vi "Update Graphs_Brass.vi"(0 "Select Graph":T8=enum."Temperature (F)", 2 "appended array":refnum<vi>[](array[refnum]), 5 "ERD Graph  Ind 2":T7, 7 "All_Bundled_Data_Brass":T1, 11 "Error In":errorcluster) -> (4 "All Loads":u16[][](graph), 12 "ERD 3":dbl(graph), 13 "ERD 2":dbl(graph), 14 "ERD 1":dbl(graph), 15 "Error Out":errorcluster)   [LabVIEW 2016]
doc: "This VI displays (makes visable) the corresponding graph based on user selection, as well as updates the values of the graphs with current data."
uses:
  type defs2/Select _Graph_Brass.ctl
  type defs2/All_Bundled_Data_Brass.ctl
  Laundry Tool 1.0 Support/type defs/Version.ctl
  type defs2/ERD_Always_Show_Brass.ctl
  type defs2/CSV_File_String_Arrays.ctl
  type defs2/Fault Table Array.ctl
  Laundry Tool 1.0 Support/type defs/Fault_Table_Info.ctl
panel:
  # "Software Version"
  # "UI"
  # "MC"
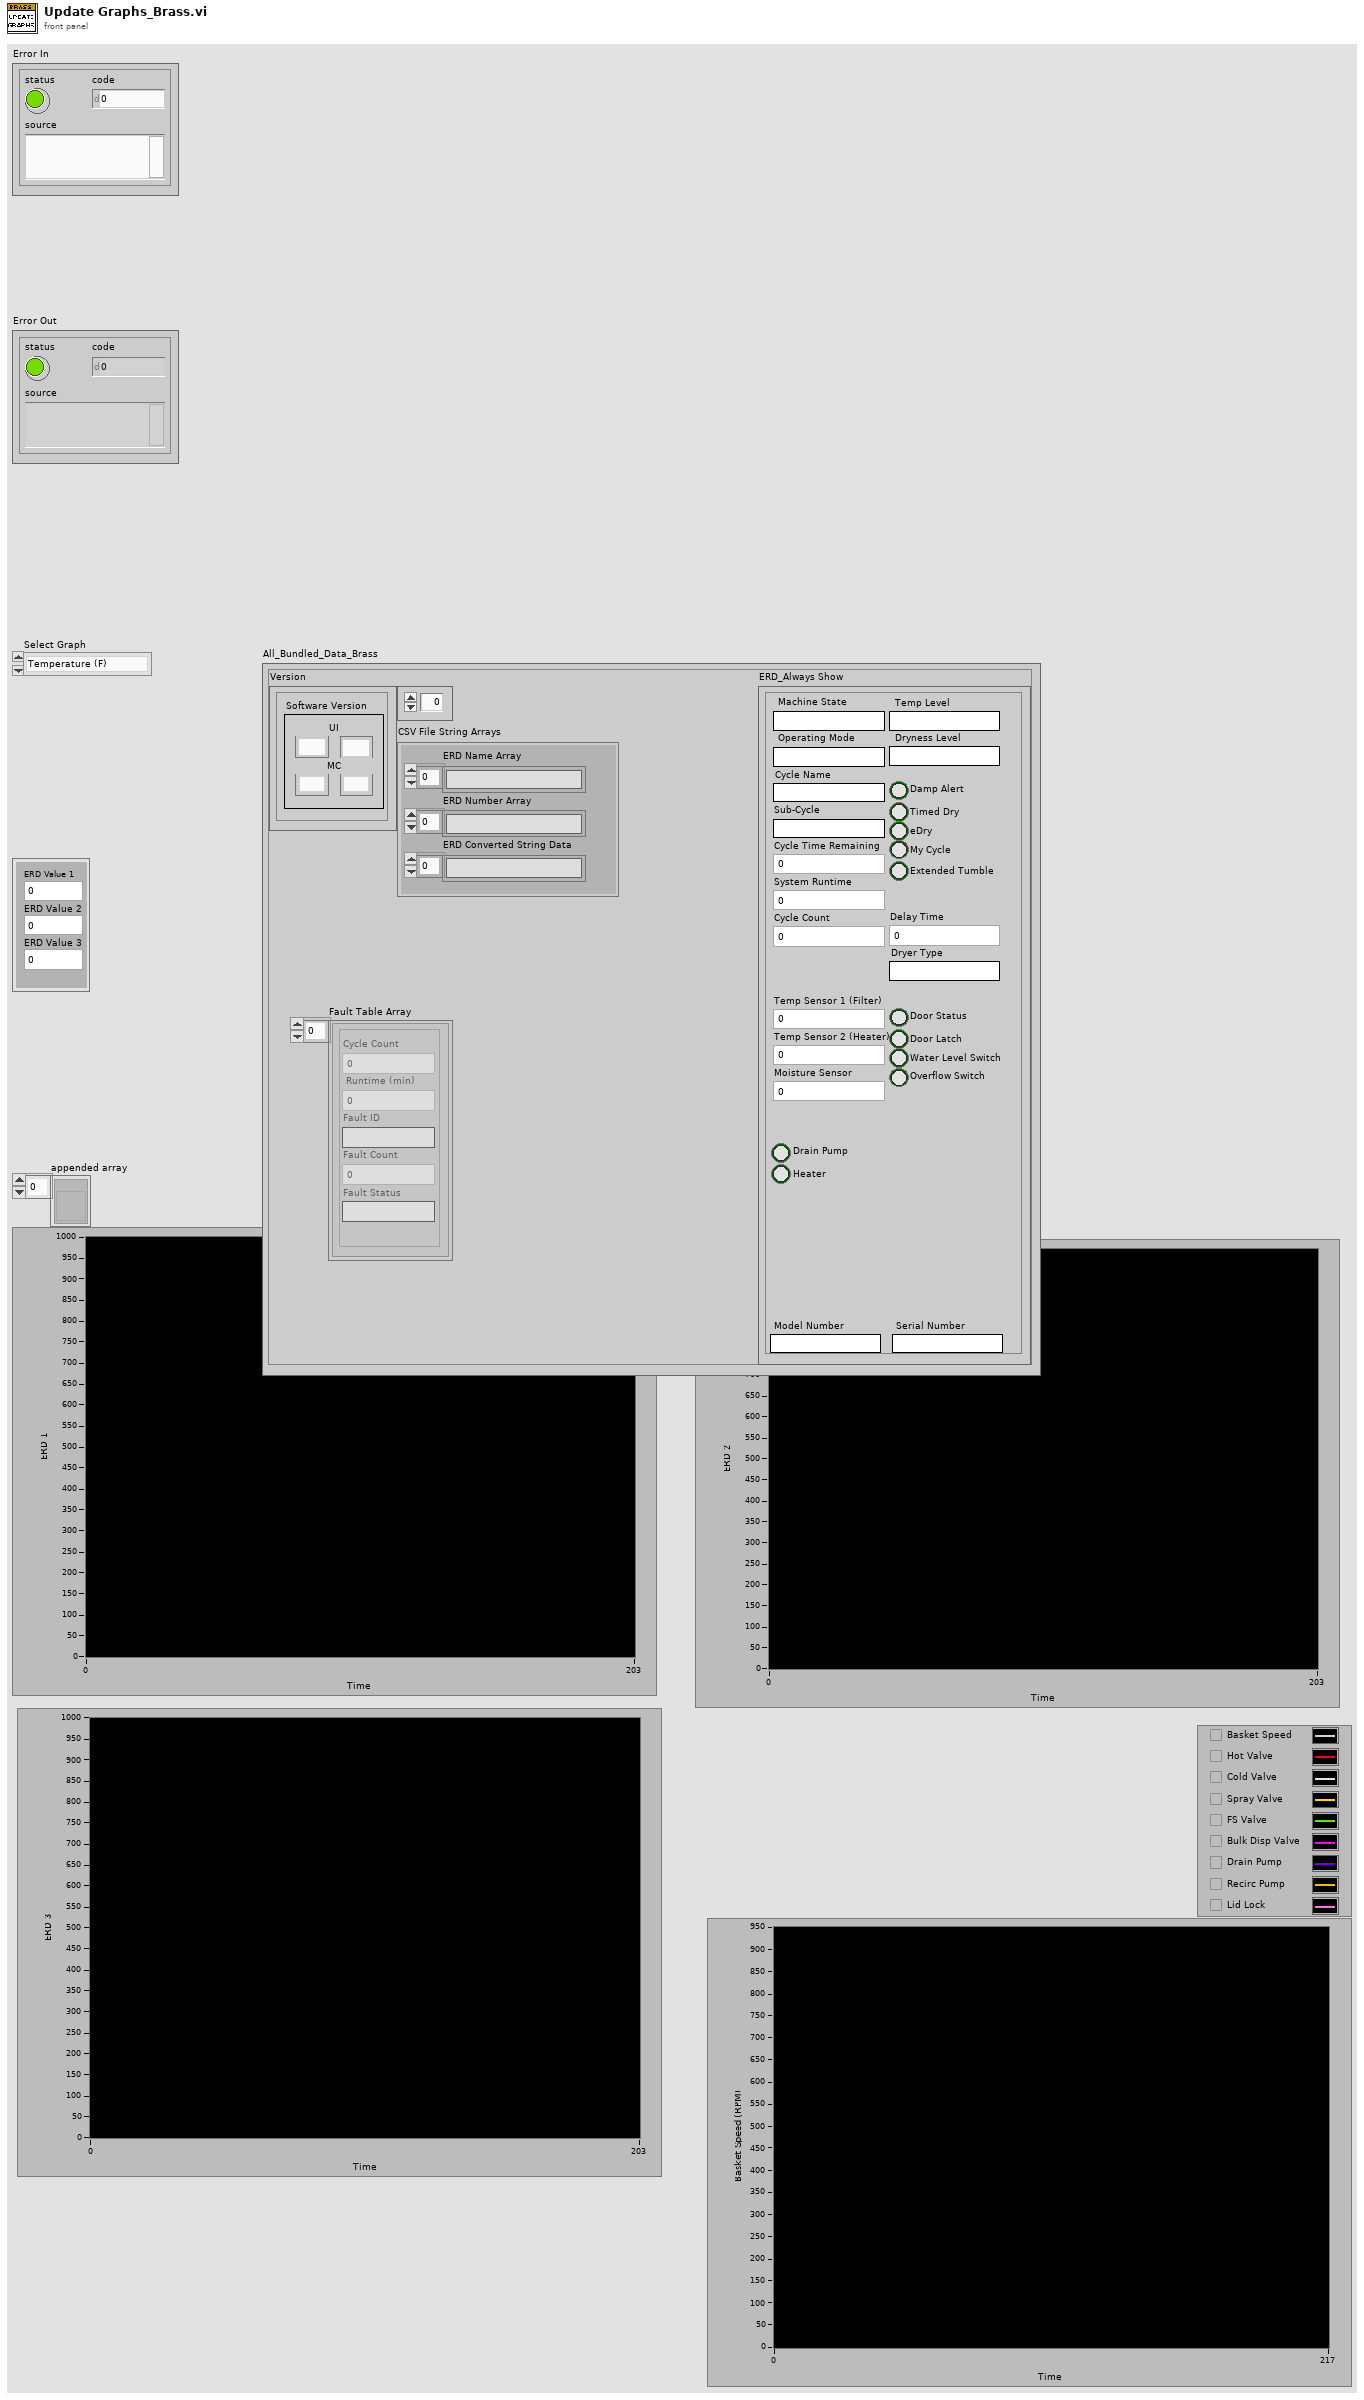
[diagram p1: front panel]
types:
  T1 = typedef "All_Bundled_Data_Brass.ctl" = cluster{"Version":T2, "ERD_Always Show":T3, "Personality Set":u8, "CSV File String Arrays":T4, "Fault Table Array ":T5}
  T2 = typedef "Version.ctl" = cluster{"Critical Major":string, "Critical Minor":string, "Non-Critical Minor":string, "Non-Critical Major":string}
  T3 = typedef "ERD_Always_Show_Brass.ctl" = cluster{"Machine State":string, "Cycle Count":u32, "Dryness Level":string, "Temp Level":string, "Delay Time":u16, "Sub-Cycle":string, "Cycle Name":string, "Model Number":string, "Serial Number":string, "System Runtime":u32, "Cycle Time Remaining":u16, "Operating Mode":string, "Temp Sensor 1 (Filter)":u16, "Drain Pump":bool, "Water Level Switch":bool, "Overflow Switch":bool, "Door Status":bool, "Door Latch":bool, "Heater":bool, "Temp Sensor 2 (Heater)":u16, "Moisture Sensor":u16, "Dryer Type":string, "eDry":bool, "Damp Alert":bool, "Timed Dry":bool, "My Cycle":bool, "Extended Tumble":bool}
  T4 = typedef "CSV_File_String_Arrays.ctl" = cluster{"ERD Number Array":string[], "ERD Name Array":string[], "ERD Converted String Data":string[]}
  T5 = typedef "Fault Table Array.ctl" = T6[]
  T6 = typedef "Fault_Table_Info.ctl" = cluster{"Cycle Count":u32, " Runtime (min) ":u32, "Fault Status":string, "Fault ID":string, "Fault Count":u16}
  T7 = cluster{"ERD Value 1":dbl, "ERD Value 2":dbl, "ERD Value 3":dbl}
  T8 = typedef "Select _Graph_Brass.ctl" = enum16{"All Loads", "ERD 1", "ERD 2", "ERD 3", "Temperature (F)", "Basket Speed (RPM)", "Tub Volume (Gal)", "Pressure (in H2O)", "Current RMS (Amps)"}
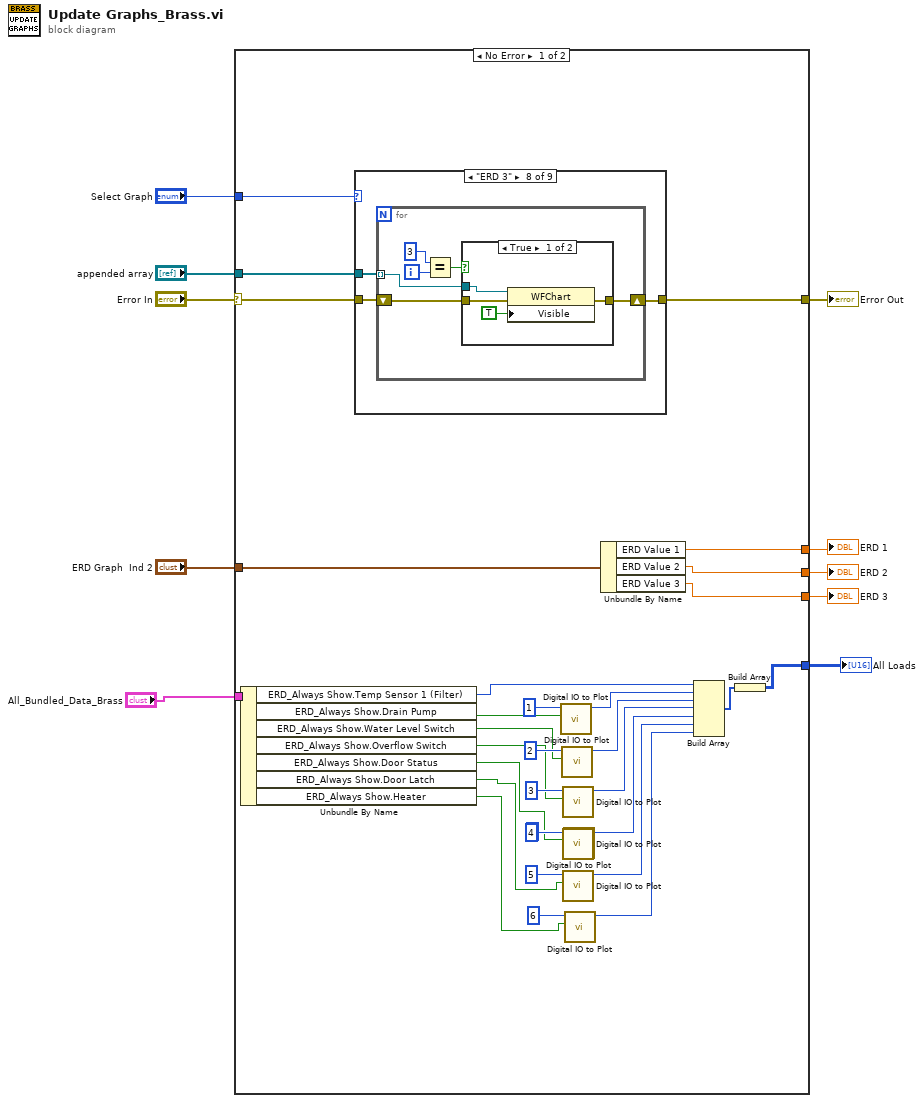
[diagram p0: block diagram]
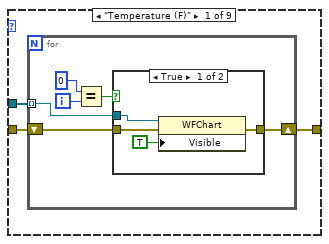
[diagram p2: hidden frame]
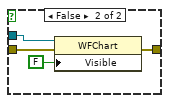
[diagram p3: hidden frame]
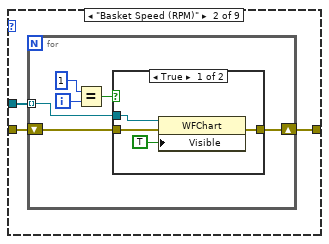
[diagram p4: hidden frame]
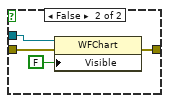
[diagram p5: hidden frame]
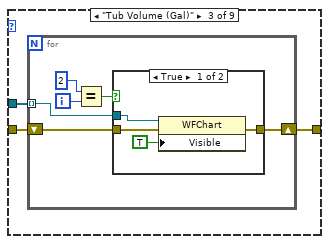
[diagram p6: hidden frame]
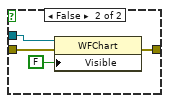
[diagram p7: hidden frame]
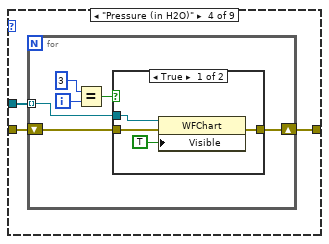
[diagram p8: hidden frame]
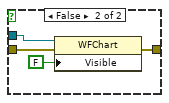
[diagram p9: hidden frame]
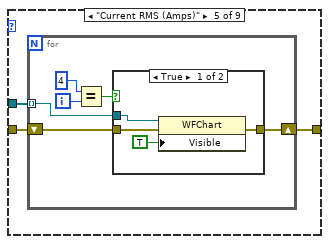
[diagram p10: hidden frame]
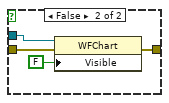
[diagram p11: hidden frame]
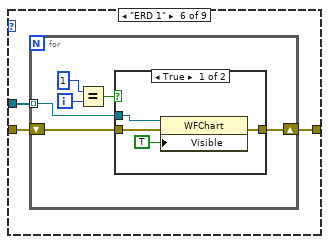
[diagram p12: hidden frame]
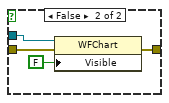
[diagram p13: hidden frame]
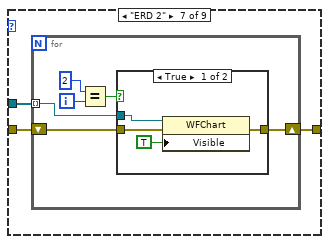
[diagram p14: hidden frame]
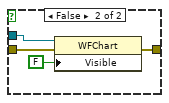
[diagram p15: hidden frame]
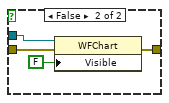
[diagram p16: hidden frame]
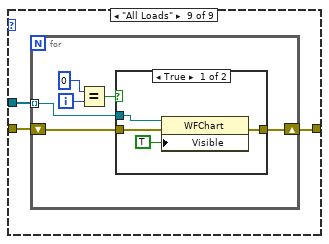
[diagram p17: hidden frame]
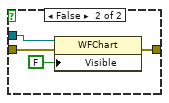
[diagram p18: hidden frame]
diagram:
  n1 = case shown="No Error" "Error In" {
    selector: "Error In" -> [w39 w195]
    tunnel: [w38 w195] -> w9
    tunnel: "appended array" -> [w40 _]
    tunnel: "Select Graph" -> [w41 _]
    tunnel: "ERD Graph  Ind 2" -> [w37 _]
    tunnel: [w36 _] -> w5
    tunnel: [w35 _] -> w4
    tunnel: [w34 _] -> w3
    tunnel: "All_Bundled_Data_Brass" -> [w33 _]
    tunnel: [w30 _] -> w2
    frame No Error {
      n2 = Unbundle By Name(w33) -> ("ERD_Always Show.Temp Sensor 1 (Filter)"=w32:u16, "ERD_Always Show.Drain Pump"=w29:bool, "ERD_Always Show.Water Level Switch"=w24:bool, "ERD_Always Show.Overflow Switch"=w23:bool, "ERD_Always Show.Door Status"=w13:bool, "ERD_Always Show.Door Latch"=w12:bool, "ERD_Always Show.Heater"=w11:bool)
      n3 = case shown="\"ERD 3\"" w41 {
        tunnel: w40 -> [w44 w61 w78 w95 w111 w128 w146 w161 w178]
        tunnel: w39 -> [w43 w60 w77 w94 w112 w129 w145 w163 w180]
        tunnel: [w42 w59 w76 w93 w110 w127 w144 w162 w179] -> w38
        frame "Temperature (F)" {
          n4 = for {
            tunnel: w44 -> [w50] mode=indexing
            shift-right: [w48] -> w42
            shift-left: w43 -> [w49]
            i -> [w47]
            n5 = Equal?(x=0 ("index"), y=w47) -> (x = y?=w45:bool)
            n6 = case shown="True" w45 {
              tunnel: w50 -> [w54 w58]
              tunnel: w49 -> [w52 w56]
              tunnel: [w51 w55] -> w48
              frame True {
                n7 = property class="WFChart"(reference=w54, error in=w52, "Visible"=TRUE) -> (error out=w51:errorcluster)  [unwired: 1 out]
              }
              frame False {
                n8 = property class="WFChart"(reference=w58, error in=w56, "Visible"=FALSE) -> (error out=w55:errorcluster)  [unwired: 1 out]
              }
            }
          }
        }
        frame "Basket Speed (RPM)" {
          n9 = for {
            tunnel: w61 -> [w67] mode=indexing
            shift-right: [w65] -> w59
            shift-left: w60 -> [w66]
            i -> [w64]
            n10 = Equal?(x=1 ("index"), y=w64) -> (x = y?=w62:bool)
            n11 = case shown="True" w62 {
              tunnel: w67 -> [w71 w75]
              tunnel: w66 -> [w69 w73]
              tunnel: [w68 w72] -> w65
              frame True {
                n12 = property class="WFChart"(reference=w71, error in=w69, "Visible"=TRUE) -> (error out=w68:errorcluster)  [unwired: 1 out]
              }
              frame False {
                n13 = property class="WFChart"(reference=w75, error in=w73, "Visible"=FALSE) -> (error out=w72:errorcluster)  [unwired: 1 out]
              }
            }
          }
        }
        frame "Tub Volume (Gal)" {
          n14 = for {
            tunnel: w78 -> [w84] mode=indexing
            shift-right: [w82] -> w76
            shift-left: w77 -> [w83]
            i -> [w81]
            n15 = Equal?(x=2 ("index"), y=w81) -> (x = y?=w79:bool)
            n16 = case shown="True" w79 {
              tunnel: w84 -> [w88 w92]
              tunnel: w83 -> [w86 w90]
              tunnel: [w85 w89] -> w82
              frame True {
                n17 = property class="WFChart"(reference=w88, error in=w86, "Visible"=TRUE) -> (error out=w85:errorcluster)  [unwired: 1 out]
              }
              frame False {
                n18 = property class="WFChart"(reference=w92, error in=w90, "Visible"=FALSE) -> (error out=w89:errorcluster)  [unwired: 1 out]
              }
            }
          }
        }
        frame "Pressure (in H2O)" {
          n19 = for {
            tunnel: w95 -> [w101] mode=indexing
            shift-right: [w99] -> w93
            shift-left: w94 -> [w100]
            i -> [w98]
            n20 = Equal?(x=3 ("index"), y=w98) -> (x = y?=w96:bool)
            n21 = case shown="True" w96 {
              tunnel: w101 -> [w105 w109]
              tunnel: w100 -> [w103 w107]
              tunnel: [w102 w106] -> w99
              frame True {
                n22 = property class="WFChart"(reference=w105, error in=w103, "Visible"=TRUE) -> (error out=w102:errorcluster)  [unwired: 1 out]
              }
              frame False {
                n23 = property class="WFChart"(reference=w109, error in=w107, "Visible"=FALSE) -> (error out=w106:errorcluster)  [unwired: 1 out]
              }
            }
          }
        }
        frame "Current RMS (Amps)" {
          n24 = for {
            tunnel: w111 -> [w118] mode=indexing
            shift-right: [w116] -> w110
            shift-left: w112 -> [w117]
            i -> [w115]
            n25 = Equal?(x=4 ("index"), y=w115) -> (x = y?=w113:bool)
            n26 = case shown="True" w113 {
              tunnel: w118 -> [w122 w126]
              tunnel: w117 -> [w120 w124]
              tunnel: [w119 w123] -> w116
              frame True {
                n27 = property class="WFChart"(reference=w122, error in=w120, "Visible"=TRUE) -> (error out=w119:errorcluster)  [unwired: 1 out]
              }
              frame False {
                n28 = property class="WFChart"(reference=w126, error in=w124, "Visible"=FALSE) -> (error out=w123:errorcluster)  [unwired: 1 out]
              }
            }
          }
        }
        frame "ERD 1" {
          n29 = for {
            tunnel: w128 -> [w135] mode=indexing
            shift-right: [w133] -> w127
            shift-left: w129 -> [w134]
            i -> [w132]
            n30 = Equal?(x=1 ("index"), y=w132) -> (x = y?=w130:bool)
            n31 = case shown="True" w130 {
              tunnel: w135 -> [w139 w143]
              tunnel: w134 -> [w137 w141]
              tunnel: [w136 w140] -> w133
              frame True {
                n32 = property class="WFChart"(reference=w139, error in=w137, "Visible"=TRUE) -> (error out=w136:errorcluster)  [unwired: 1 out]
              }
              frame False {
                n33 = property class="WFChart"(reference=w143, error in=w141, "Visible"=FALSE) -> (error out=w140:errorcluster)  [unwired: 1 out]
              }
            }
          }
        }
        frame "ERD 2" {
          n34 = for {
            tunnel: w146 -> [w152] mode=indexing
            shift-right: [w150] -> w144
            shift-left: w145 -> [w151]
            i -> [w149]
            n35 = Equal?(x=2 ("index"), y=w149) -> (x = y?=w147:bool)
            n36 = case shown="True" w147 {
              tunnel: w152 -> [w156 w160]
              tunnel: w151 -> [w154 w158]
              tunnel: [w153 w157] -> w150
              frame True {
                n37 = property class="WFChart"(reference=w156, error in=w154, "Visible"=TRUE) -> (error out=w153:errorcluster)  [unwired: 1 out]
              }
              frame False {
                n38 = property class="WFChart"(reference=w160, error in=w158, "Visible"=FALSE) -> (error out=w157:errorcluster)  [unwired: 1 out]
              }
            }
          }
        }
        frame "ERD 3" {
          n39 = for {
            tunnel: w161 -> [w169] mode=indexing
            shift-right: [w167] -> w162
            shift-left: w163 -> [w168]
            i -> [w166]
            n40 = Equal?(x=3 ("index"), y=w166) -> (x = y?=w164:bool)
            n41 = case shown="True" w164 {
              tunnel: w169 -> [w173 w177]
              tunnel: w168 -> [w171 w175]
              tunnel: [w170 w174] -> w167
              frame True {
                n42 = property class="WFChart"(reference=w173, error in=w171, "Visible"=TRUE) -> (error out=w170:errorcluster)  [unwired: 1 out]
              }
              frame False {
                n43 = property class="WFChart"(reference=w177, error in=w175, "Visible"=FALSE) -> (error out=w174:errorcluster)  [unwired: 1 out]
              }
            }
          }
        }
        frame "All Loads" {
          n44 = for {
            tunnel: w178 -> [w186] mode=indexing
            shift-right: [w184] -> w179
            shift-left: w180 -> [w185]
            i -> [w183]
            n45 = Equal?(x=0 ("index"), y=w183) -> (x = y?=w181:bool)
            n46 = case shown="True" w181 {
              tunnel: w186 -> [w190 w194]
              tunnel: w185 -> [w188 w192]
              tunnel: [w187 w191] -> w184
              frame True {
                n47 = property class="WFChart"(reference=w190, error in=w188, "Visible"=TRUE) -> (error out=w187:errorcluster)  [unwired: 1 out]
              }
              frame False {
                n48 = property class="WFChart"(reference=w194, error in=w192, "Visible"=FALSE) -> (error out=w191:errorcluster)  [unwired: 1 out]
              }
            }
          }
        }
      }
      n49 = call "Digital IO to Plot.vi"("Boolean Value"=w29, "Multiplier"=u16 1) -> ("Output"=w22:u16)  [unwired: 9 in]
      n50 = call "Digital IO to Plot.vi"("Boolean Value"=w24, "Multiplier"=u16 2) -> ("Output"=w21:u16)  [unwired: 9 in]
      n51 = call "Digital IO to Plot.vi"("Boolean Value"=w23, "Multiplier"=u16 3) -> ("Output"=w20:u16)  [unwired: 9 in]
      n52 = call "Digital IO to Plot.vi"("Multiplier"=u16 4) -> ("Output"=w19:u16)  [unwired: 10 in]
      n53 = call "Digital IO to Plot.vi"("Boolean Value"=w12, "Multiplier"=u16 5) -> ("Output"=w15:u16)  [unwired: 9 in]
      n54 = call "Digital IO to Plot.vi"("Boolean Value"=w13, "Multiplier"=u16 4) -> ()  [unwired: 9 in, 1 out]
      n55 = call "Digital IO to Plot.vi"("Boolean Value"=w11, "Multiplier"=u16 6) -> ("Output"=w14:u16)  [unwired: 9 in]
      n56 = Unbundle By Name(w37) -> ("ERD Value 1"=w36:dbl, "ERD Value 2"=w35:dbl, "ERD Value 3"=w34:dbl)
      n57 = Build Array(w32, w22, w21, w20, w19, w15, w14) -> (w31:u16[])
      n58 = Build Array(w31) -> (w30:u16[][])
    }
    frame Error {
    }
  }
  "Error Out" <- w9
  "ERD 1" <- w5
  "ERD 2" <- w4
  "ERD 3" <- w3
  "All Loads" <- w2
